vi "Change DocumentTag.vi"(8 "error in (no error)":errorcluster, 9 "Copy Help Tag":bool, 10 "Help.Tag":string, 11 "Help:Document Tag W":refnum<vi>) -> (0 "error out":errorcluster)   [LabVIEW 2020]
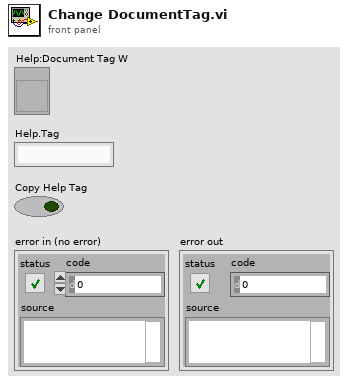
[diagram p1: front panel]
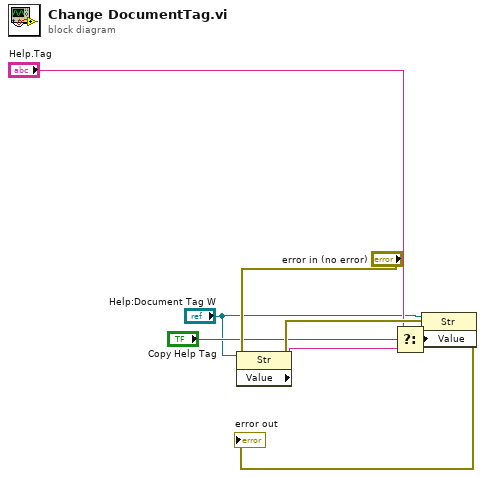
[diagram p0: block diagram]
diagram:
  n1 = property on="Property Node" class="Str"(reference="Help:Document Tag W", error in="error in (no error)") -> (error out=w7:errorcluster, "Value"=w5:string)  [unwired: 1 out]
  n2 = Select(t="Help.Tag", s="Copy Help Tag", f=w5) -> (s? t:f=w2:string)
  n3 = property on="Property Node" class="Str"(reference="Help:Document Tag W", error in=w7, "Value"=w2) -> (error out=→"error out":errorcluster)  [unwired: 1 out]
